vi "Write Image.vi"(8 "error in (no error)":errorcluster, 9 "2D Picture":picture, 11 "64x128 I2C OLED SSD1315 In":refnum<class "64x128 I2C OLED SSD1315.lvclass">) -> (0 "error out":errorcluster, 3 "64x128 I2C OLED SSD1315 Out":refnum<class "64x128 I2C OLED SSD1315.lvclass">)   [LabVIEW 2020, in "CTI-Peripheral.lvlib" / "64x128 I2C OLED SSD1315.lvclass"]
uses:
  64x128 I2C OLED SSD1315.lvclass
  64x128 I2C OLED SSD1315.lvclass/64x128 I2C OLED SSD1315.ctl
  CTI/I2C Connection/I2C Connection.lvclass/I2C Connection.ctl
  Private/BuildMessagesFromPicture.vi
  CTI/Session/I2C Write Data.vi
  CTI/I2C Connection/I2C Connection.lvclass
panel:
  out "Generate":dbl
  out "Write":dbl
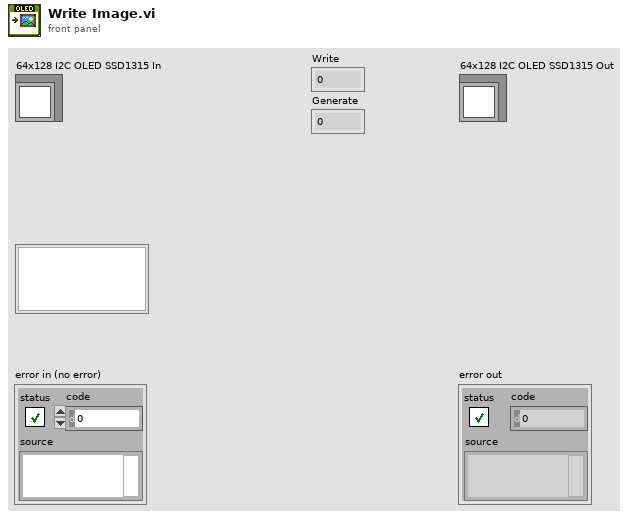
[diagram p1: front panel]
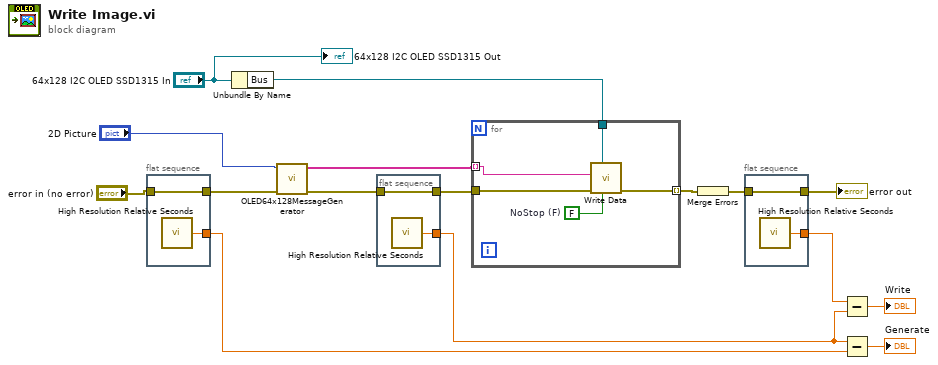
[diagram p0: block diagram]
diagram:
  n1 = flat-sequence {
    tunnel: "error in (no error)" -> [w18]
    tunnel: [w18] -> w8
    tunnel: [w17] -> w5
    frame #0 {
      n2 = call <vilib>:"High Resolution Relative Seconds.vi"() -> ("relative seconds"=w17:dbl)
    }
  }
  n3 = Unbundle By Name("64x128 I2C OLED SSD1315 In") -> ("Bus"=w14:refnum<class "I2C Connection.lvclass">)
  n4 = call-poly "OLED64x128MessageGenerator.vi"("error in (no error)"=w8, "2D Picture"="2D Picture") -> ("error out"=w11:errorcluster, "Messages"=w16:string[])  [unwired: 8 in]
  n5 = flat-sequence {
    tunnel: w11 -> [w20]
    tunnel: [w20] -> w10
    tunnel: [w19] -> w3
    frame #0 {
      n6 = call <vilib>:"High Resolution Relative Seconds.vi"() -> ("relative seconds"=w19:dbl)
    }
  }
  n7 = for {
    tunnel: w14 -> [w24]
    tunnel: w16 -> [w21] mode=indexing
    tunnel: w10 -> [w22]
    tunnel: [w25] -> w12 mode=indexing
    w23 = FALSE  # NoStop (F)
    n8 = call "Write Data.vi"("NoStop (F)"=w23, "I2C Connection"=w24, "error in (no error)"=w22, "Data"=w21) -> ("error out"=w25:errorcluster)  [unwired: 7 in]
  }
  n9 = Merge Errors(w12) -> (w7:errorcluster)
  n10 = flat-sequence {
    tunnel: w7 -> [w27]
    tunnel: [w27] -> w6
    tunnel: [w26] -> w4
    frame #0 {
      n11 = call <vilib>:"High Resolution Relative Seconds.vi"() -> ("relative seconds"=w26:dbl)
    }
  }
  n12 = Subtract(x=w4, y=w3) -> (x-y=→"Write":dbl)
  n13 = Subtract(x=w3, y=w5) -> (x-y=→"Generate":dbl)
  "error out" <- w6
  "64x128 I2C OLED SSD1315 Out" <- "64x128 I2C OLED SSD1315 In"
